vi "To Pretty String (Boolean).vi"(8 "error in (no error)":errorcluster, 10 "indent":i32, 11 "JSON Value in":variant) -> (0 "error out":errorcluster, 3 "String":string)   [LabVIEW 2017, in "JSON Support for LabVIEW.lvlib"]
uses:
  JSON Support for LabVIEW.lvlib
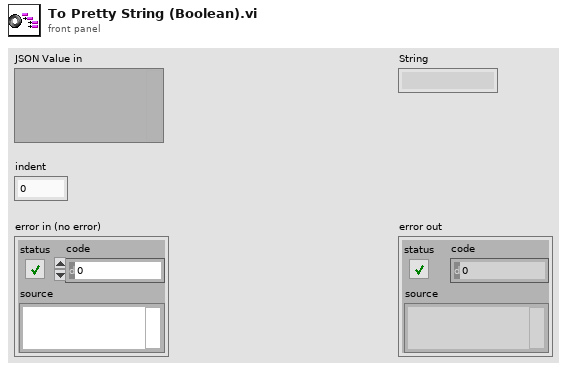
[diagram p1: front panel]
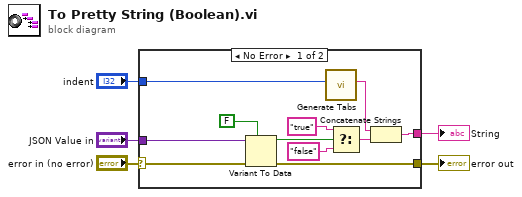
[diagram p0: block diagram]
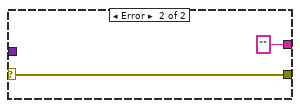
[diagram p2: hidden frame]
diagram:
  n1 = case shown="No Error" "error in (no error)" {
    selector: "error in (no error)" -> [w12 w17]
    tunnel: "JSON Value in" -> [w16 _]
    tunnel: [w6 "" ("f")] -> w4
    tunnel: [w11 w17] -> w2
    tunnel: "indent" -> [w9 _]
    frame No Error {
      n2 = Variant To Data(error in=w12, type=FALSE, Variant=w16) -> (data=w10:bool, error out=w11:errorcluster)
      n3 = call "Generate Tabs.vi"("indent"=w9) -> ("Tabs"=w8:string)  [unwired: 9 in, 1 out]
      n4 = Select(t="true" ("String"), s=w10, f="false") -> (s? t:f=w7:string)
      n5 = Concatenate Strings(w8, w7) -> (w6:string)
    }
    frame Error {
    }
  }
  "String" <- w4
  "error out" <- w2
